vi "Read Channels for gRPC.vi"(11 "CIFCorePlugin in":refnum<class "CIFCorePlugin.lvclass">) -> (3 "Channels":T1[](array[typedef]))   [LabVIEW 2021, in "CIFCorePlugin.lvclass"]
uses:
  CIFCorePlugin.lvclass
  CIFCorePlugin.lvclass/CIFCorePlugin.ctl
  Channels/CIFChannelMng/CIFChannelMng.lvclass
  Grpc/CIFCoreChannel_server/RPC Messages/cif_channelcore_ChannelPattern.ctl
  Grpc/CIFCoreChannel_server/CIFCoreChannel_server.lvlib
  Grpc/CIFCoreChannel_server/RPC Messages/cif_channelcore_ChannelDirection.ctl
  Grpc/CIFCoreChannel_server/RPC Messages/cif_channelcore_Channel.ctl
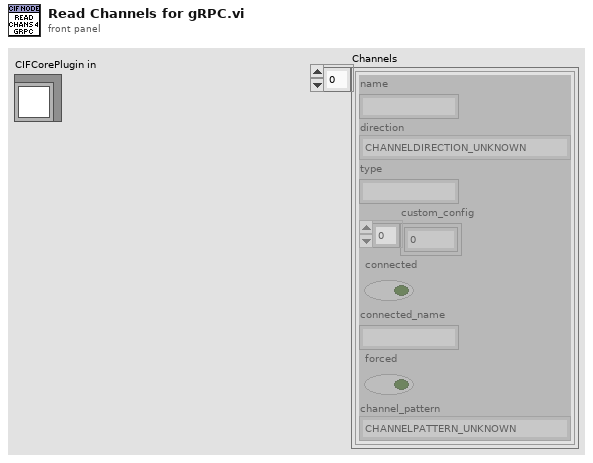
[diagram p1: front panel]
types:
  T1 = typedef "CIFCoreChannel_server.lvlib/cif_channelcore_Channel.ctl" = cluster{"name":string, "direction":T2, "type":string, "custom_config":u8[], "connected":bool, "connected_name":string, "forced":bool, "channel_pattern":T3}
  T2 = typedef "CIFCoreChannel_server.lvlib/cif_channelcore_ChannelDirection.ctl" = enum32{"CHANNELDIRECTION_UNKNOWN", "CHANNELDIRECTION_PUBLISHER", "CHANNELDIRECTION_SUBSCRIBER"}
  T3 = typedef "CIFCoreChannel_server.lvlib/cif_channelcore_ChannelPattern.ctl" = enum32{"CHANNELPATTERN_UNKNOWN", "CHANNELPATTERN_TAG", "CHANNELPATTERN_FIFO", "CHANNELPATTERN_MULTIFIFO", "CHANNELPATTERN_BACKPRESSUREFIFO"}
  T4 = typedef "CIFChannelMng.lvclass/Channel List for OOB.ctl" = cluster{"Name":string, "Direction":T5, "Type":string, "Connected?":bool, "Connected Name":string, "Custom Config Data":u8[], "Forced?":bool, "Pattern":T6}
  T5 = typedef "CIFChannels.lvclass/Direction.ctl" = enum16{"Publisher", "Subscriber"}
  T6 = typedef "ChannelCommon.lvlib/Channel Pattern.ctl" = enum16{"Unknown", "Tag", "FIFO", "MultiFIFO", "BackpressureFIFO"}
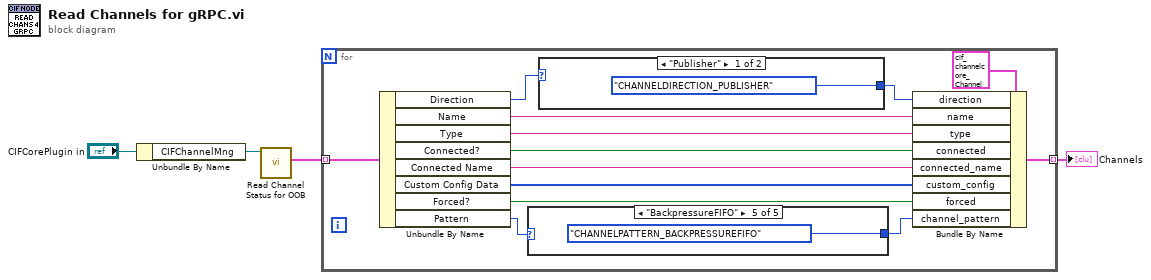
[diagram p0: block diagram]
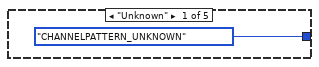
[diagram p2: hidden frame]
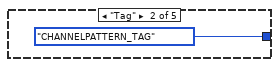
[diagram p3: hidden frame]
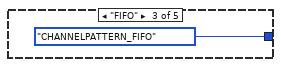
[diagram p4: hidden frame]
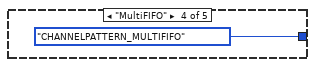
[diagram p5: hidden frame]
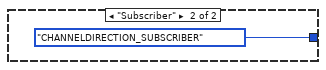
[diagram p6: hidden frame]
diagram:
  n1 = Unbundle By Name("CIFCorePlugin in") -> ("CIFChannelMng"=w4:refnum<class "CIFChannelMng.lvclass">)
  n2 = call "Read Channel Status for OOB.vi"("CIFChannelMng in"=w4) -> ("Channel Status for OOB"=w3:T4[])  [unwired: 8 in, 2 out]
  n3 = for {
    tunnel: w3 -> [w17] mode=indexing
    tunnel: [w11] -> w1 mode=indexing
    n4 = Unbundle By Name(w17) -> ("Direction"=w6:T5, "Name"=w15:string, "Type"=w14:string, "Connected?"=w13:bool, "Connected Name"=w12:string, "Custom Config Data"=w10:u8[], "Forced?"=w9:bool, "Pattern"=w7:T6)
    n5 = case shown="\"BackpressureFIFO\"" w7 {
      tunnel: [cif_channelcore_ChannelPattern."CHANNELPATTERN_UNKNOWN" ("channel_pattern") cif_channelcore_ChannelPattern."CHANNELPATTERN_TAG" ("channel_pattern") cif_channelcore_ChannelPattern."CHANNELPATTERN_FIFO" ("channel_pattern") cif_channelcore_ChannelPattern."CHANNELPATTERN_MULTIFIFO" ("channel_pattern") cif_channelcore_ChannelPattern."CHANNELPATTERN_BACKPRESSUREFIFO" ("channel_pattern")] -> w8
      frame "Unknown" {
      }
      frame "Tag" {
      }
      frame "FIFO" {
      }
      frame "MultiFIFO" {
      }
      frame "BackpressureFIFO" {
      }
    }
    n6 = case shown="\"Publisher\"" w6 {
      tunnel: [cif_channelcore_ChannelDirection."CHANNELDIRECTION_PUBLISHER" ("direction") cif_channelcore_ChannelDirection."CHANNELDIRECTION_SUBSCRIBER" ("direction")] -> w5
      frame "Publisher" {
      }
      frame "Subscriber" {
      }
    }
    n7 = Bundle By Name(cluster=T1 {"name"="", "direction"=enum."CHANNELDIRECTION_UNKNOWN", "type"="", "custom_config"=[], "connected"=FALSE, "connected_name"="", "forced"=FALSE, "channel_pattern"=enum."CHANNELPATTERN_UNKNOWN"} ("cif_channelcore_Channel"), "direction"=w5, "name"=w15, "type"=w14, "connected"=w13, "connected_name"=w12, "custom_config"=w10, "forced"=w9, "channel_pattern"=w8) -> (w11:T1)
  }
  "Channels" <- w1
